vi "PC Main.vi"() -> ()   [LabVIEW 2018]
uses:
  <vilib>/Utility/inputDevices.llb/joystickAcquire.vi
  <vilib>/Utility/inputDevices.llb/closeJoystick.vi
  <resource>/objmgr/ni.dex.rc
panel:
  in  "myRIO IP address":string(combo)
  out "ScaledValues 2":dbl[](array[numeric])
  out "timed out?":bool
  in  "Stop Button":bool
  out "RT reader URL":string="//10.99.99.109/RT-reader"
  out "RT connected?":bool=TRUE
  out "error out 2":errorcluster
  out "direction info 3":T1={"pov 1"=-1, "pov 2"=-1, "pov 3"=-1, "pov 4"=-1}
  in  "stop 2":bool
  out "axis info 2":T2
  out "Angular Velocity":dbl
  out "Y velocity":dbl
  out "X velocity":dbl
  out "error out":errorcluster
  out "direction info 2":T1={"pov 1"=-1, "pov 2"=-1, "pov 3"=-1, "pov 4"=-1}
  in  "stop":bool
  out "array":i32[](array[numeric])=[289, 1907, -32768, 34, 2313, -32768, 0, 0]
  in  "LeftStick Deadzone -":dbl
  in  "LeftStick Deadzone +":dbl=2700.0
  in  "RightStick Deadzone -":dbl=-250.0
  in  "RightStick Deadzone +":dbl=2000.0
  out "LeftStick":dbl
  out "RightStick":dbl
  out "LeftOutput+":dbl
  out "LeftOutput-":dbl
  out "RightOutput+":dbl
  out "RightOutput-":dbl
  out "ScaledValues":dbl[](array[numeric])
  # "PC host writer"
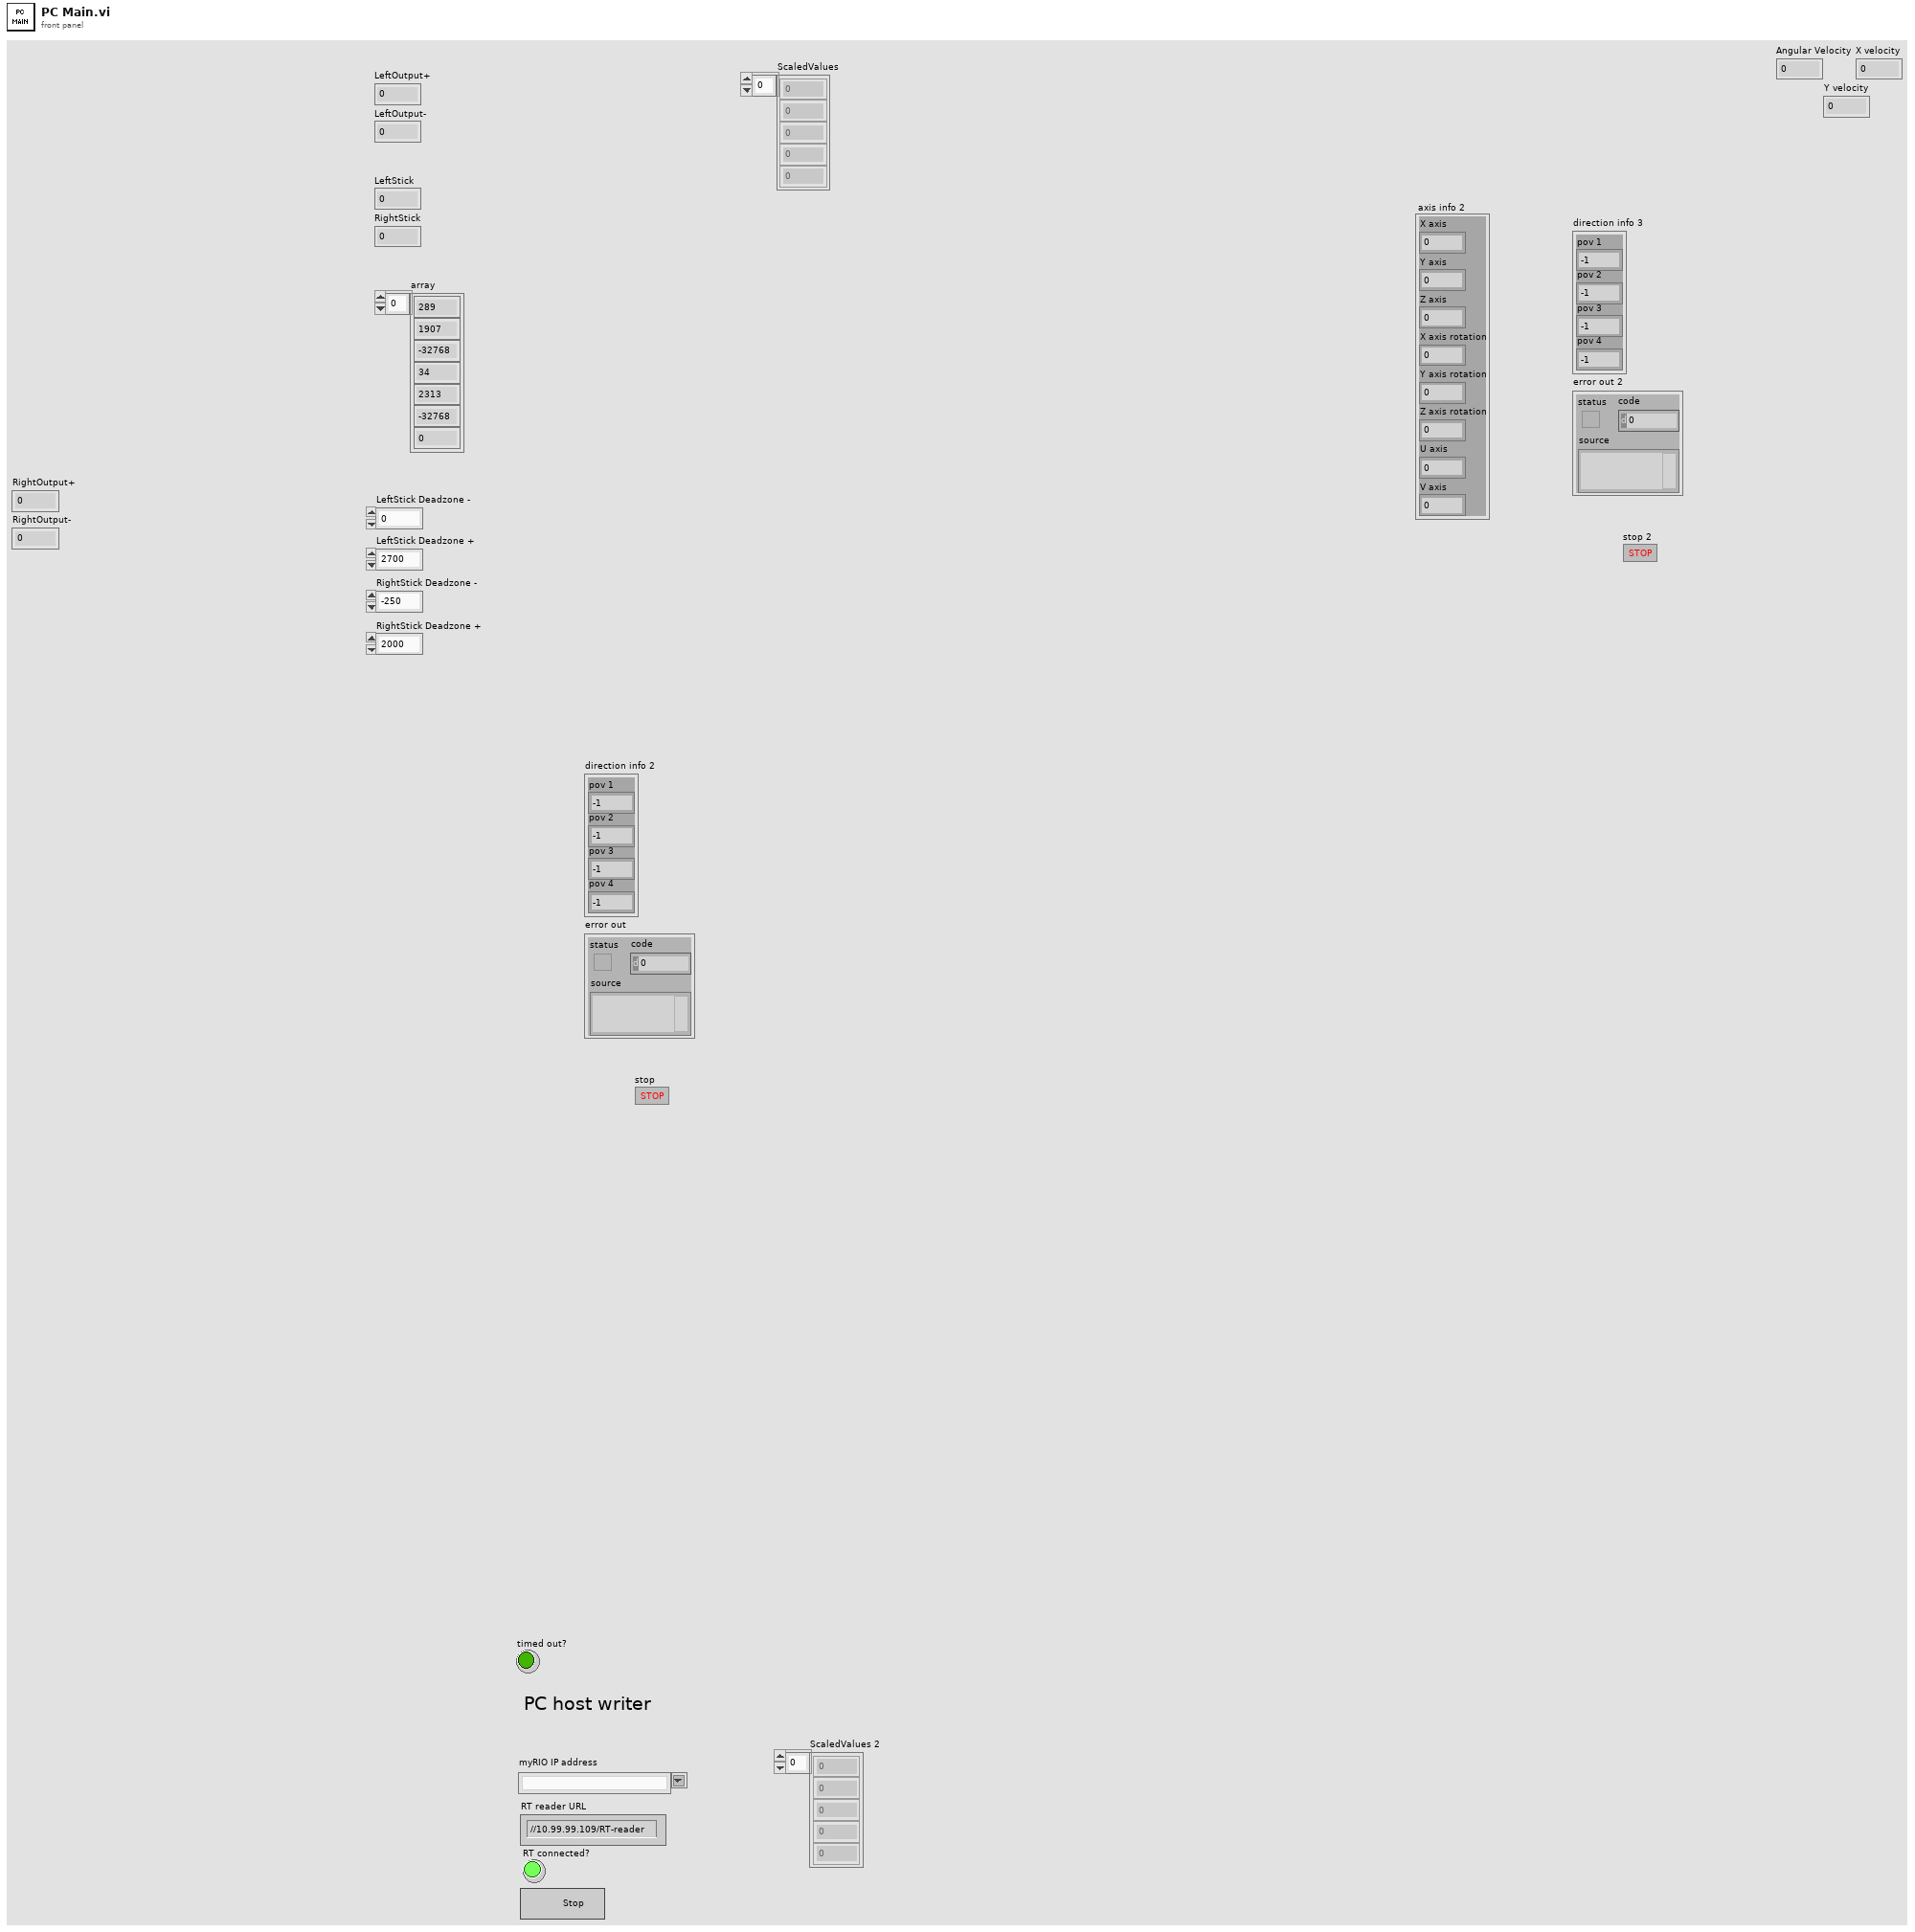
[diagram p1: front panel]
types:
  T1 = cluster{"pov 1":i32, "pov 2":i32, "pov 3":i32, "pov 4":i32}
  T2 = cluster{"X axis":i32, "Y axis":i32, "Z axis":i32, "X axis rotation":i32, "Y axis rotation":i32, "Z axis rotation":i32, "U axis":i32, "V axis":i32}
  T3 = cluster{"button 1":bool, "button 2":bool, "button 3":bool, "button 4":bool, "button 5":bool, "button 6":bool, "button 7":bool, "button 8":bool, "button 9":bool, "button 10":bool, "button 11":bool, "button 12":bool, "button 13":bool, "button 14":bool, "button 15":bool, "button 16":bool, "button 17":bool, "button 18":bool, "button 19":bool, "button 20":bool, "button 21":bool, "button 22":bool, "button 23":bool, "button 24":bool, "button 25":bool, "button 26":bool, "button 27":bool, "button 28":bool, "button 29":bool, "button 30":bool, "button 31":bool, "button 32":bool}
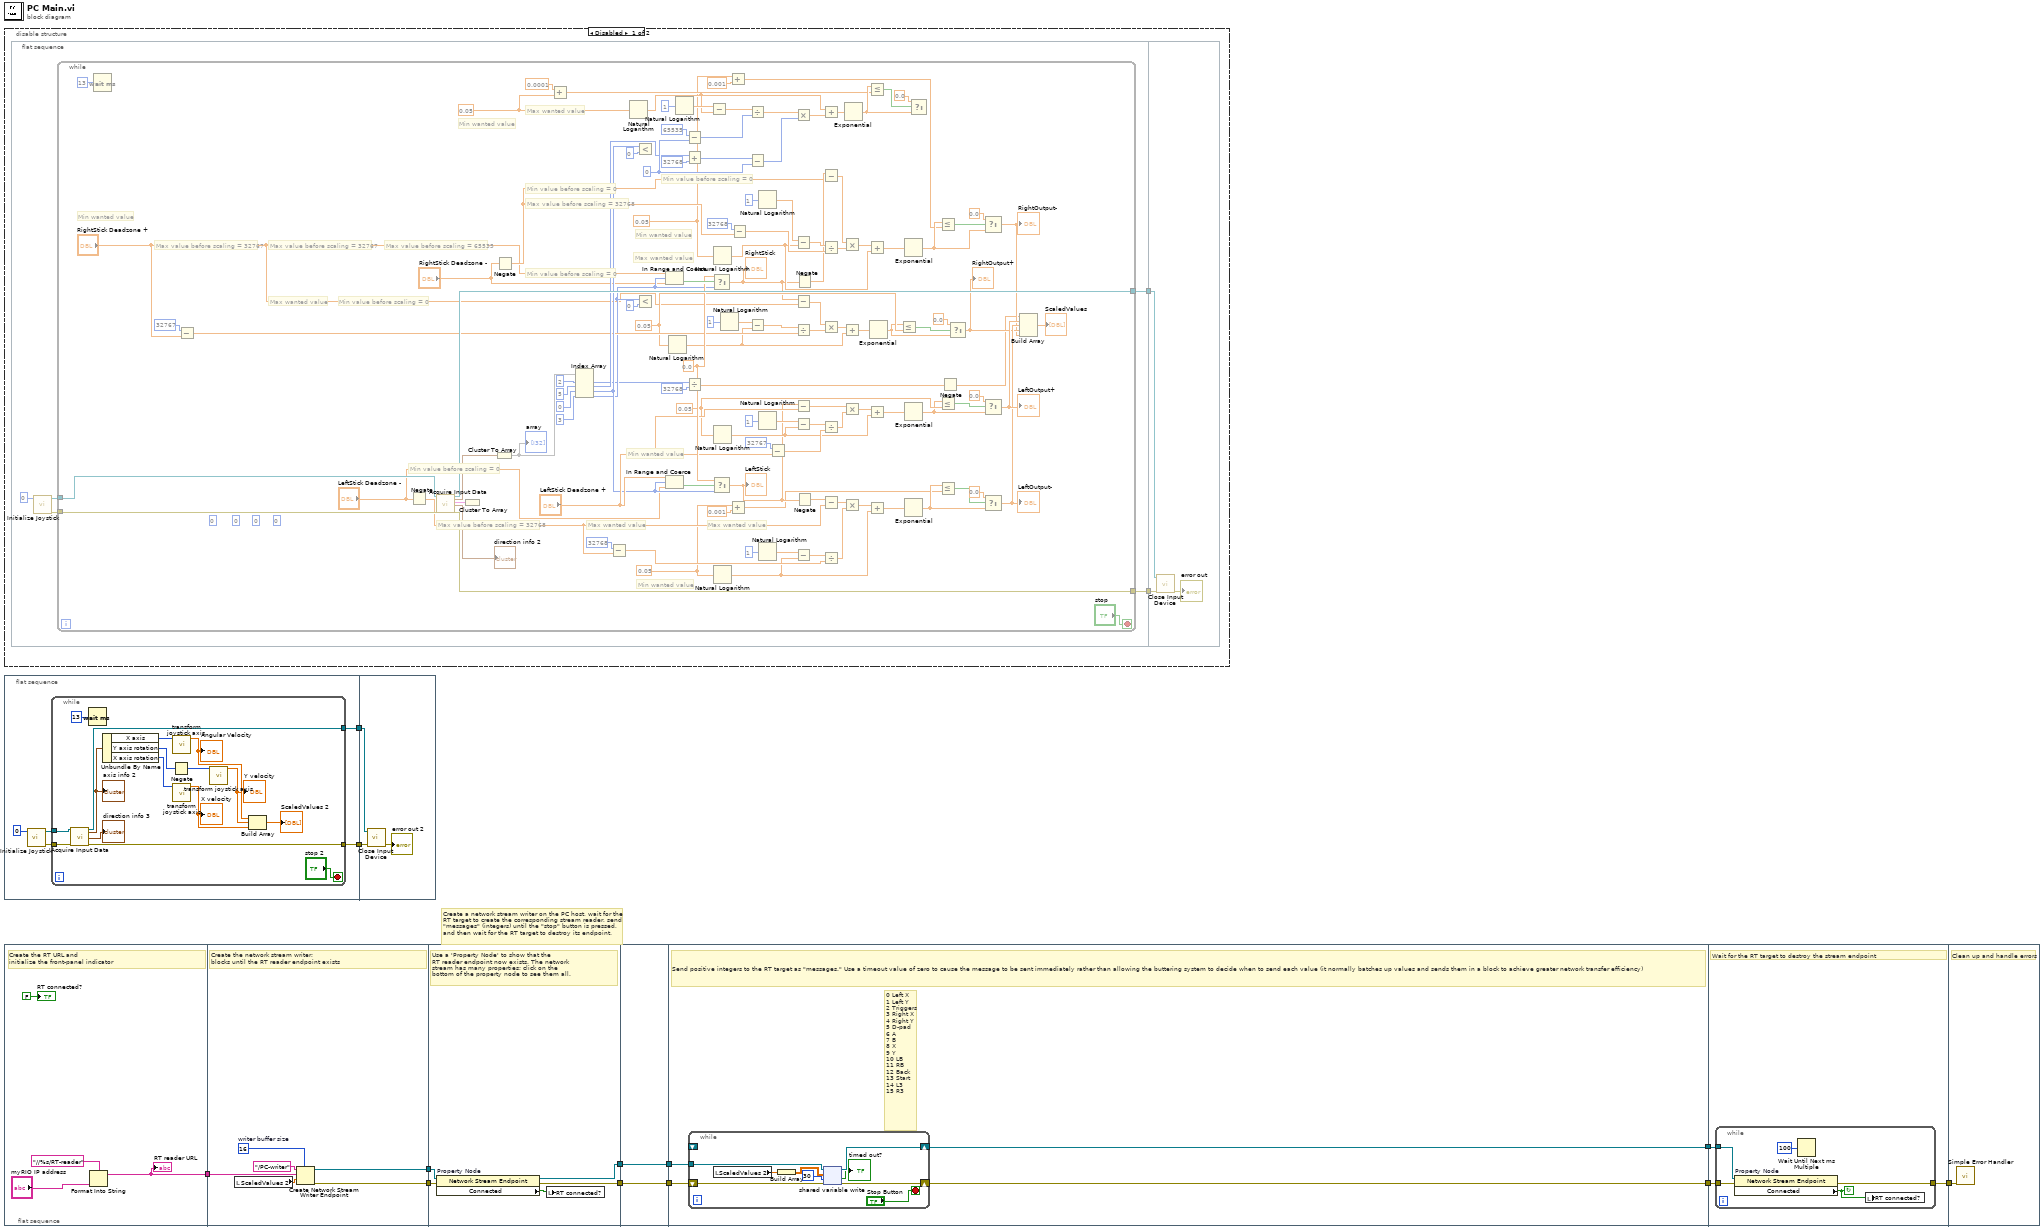
[diagram p0: block diagram]
diagram:
  # "Create a network stream writer on the PC host, wait for the\nRT target to create the corresponding stream reader, send\n\"messages\" (integers) until the \"stop\" button is pressed,\nand then wait for the RT target to destroy its endpoint."
  n1 = disable-structure shown="Disabled" {
    frame Disabled {
      n2 = flat-sequence {
        tunnel: [w17] -> w14
        tunnel: [w16] -> w13
        tunnel: w14 -> [w142]
        tunnel: w13 -> [w141]
        frame #0 {
          n3 = call <vilib>:"Initialize Joystick.vi"("device index"=0) -> ("error out"=w18:errorcluster, "device ID"=w19:refnum<k1>)  [unwired: 9 in]
          n4 = while {
            tunnel: w19 -> [w138]
            tunnel: w18 -> [w137]
            tunnel: [w136] -> w17
            tunnel: [w134] -> w16
            stop <- "stop" stop-if-true
            w35 = 0.05 ("x")
            (unwired) 0 ("index")
            w55 = 0.05 ("x")
            (unwired) 0 ("index")
            w68 = 0.05 ("x")
            (unwired) 0 ("index")
            w91 = 0.05 ("x")
            (unwired) 0 ("index")
            w103 = 0.0 ("t")
            w110 = 0.05 ("x")
            w124 = 0 ("index")
            # "Min wanted value"
            # "Max wanted value"
            # "Max value before scaling = 32768"
            # "Min value before scaling = 0"
            # "Min wanted value"
            # "Max wanted value"
            # "Max value before scaling = 32767"
            # "Min value before scaling = 0"
            # "Min wanted value"
            # "Max wanted value"
            # "Max value before scaling = 32768"
            # "Min value before scaling = 0"
            # "Min wanted value"
            # "Max wanted value"
            # "Max value before scaling = 32767"
            # "Min value before scaling = 0"
            # "Min wanted value"
            # "Max wanted value"
            # "Max value before scaling = 65535"
            # "Min value before scaling = 0"
            n5 = Wait (ms)(milliseconds to wait=u32 13) -> ()  [unwired: 1 out]
            n6 = Subtract(x=32767 ("index"), y="RightStick Deadzone +") -> (x-y=w61:dbl)
            n7 = Negate(x="LeftStick Deadzone -") -> (-x=w69:dbl)
            n8 = call-poly <vilib>:"Acquire Input Data.vi"("device ID"=w138, "error in (no error)"=w137) -> ("device ID"=w136:refnum<k1>, "axis info"=w133:T2, "button info"=w132:T3, "direction info"=→"direction info 2":T1, "error out"=w134:errorcluster)  [unwired: 13 in]
            n9 = Cluster To Array(cluster=w132) -> ()  [unwired: 1 out]
            n10 = Cluster To Array(cluster=w133) -> (array=w131:i32[])
            "array" <- w131
            n11 = Negate(x="RightStick Deadzone -") -> (-x=w36:dbl)
            n12 = Add(x=0.0001 ("y"), y=w110) -> (x+y=w108:dbl)
            n13 = Index Array(array=w131, index #1=2 ("index"), index #2=5 ("index"), index #3=0 ("index"), index #4=3 ("index")) -> (element #1=w22:i32, element #2=w116:i32, element #3=w73:i32, element #4=w32:i32)
            n14 = Subtract(x=32768 ("index"), y=w69) -> (x-y=w82:dbl)
            n15 = Natural Logarithm(1:w110) -> (0:w120:dbl)
            n16 = Less?(x=w73, y=0) -> ()  [unwired: 1 out]
            n17 = Less?(x=w32, y=0) -> ()  [unwired: 1 out]
            n18 = In Range and Coerce(upper limit="RightStick Deadzone +", x=w32, lower limit="RightStick Deadzone -") -> (In Range?=w105:bool)  [unwired: 1 out]
            n19 = In Range and Coerce(upper limit="LeftStick Deadzone +", x=w73, lower limit="LeftStick Deadzone -") -> (In Range?=w104:bool)  [unwired: 1 out]
            n20 = Natural Logarithm(1:w55) -> (0:w57:dbl)
            n21 = Natural Logarithm(1:1 ("index")) -> (0:w128:dbl)
            n22 = Subtract(x=65535 ("index"), y=w124) -> (x-y=w125:i32)
            n23 = Add(x=w116, y=32768) -> (x+y=w115:i32)
            n24 = Divide(x=w22, y=32768) -> (x/y=w21:dbl)
            n25 = Subtract(x=w128, y=w120) -> (x-y=w127:dbl)
            n26 = Select(t=w103, s=w105, f=w32) -> (s? t:f=w31:dbl)
            "RightStick" <- w31
            n27 = Select(t=w103, s=w104, f=w73) -> (s? t:f=w72:dbl)
            "LeftStick" <- w72
            n28 = Natural Logarithm(1:w35) -> (0:w42:dbl)
            n29 = Natural Logarithm(1:w91) -> (0:w93:dbl)
            n30 = Natural Logarithm(1:w68) -> (0:w78:dbl)
            n31 = Natural Logarithm(1:1 ("index")) -> (0:w63:dbl)
            n32 = Add(x=w35, y=0.001) -> (x+y=w33:dbl)
            n33 = Add(x=w68, y=0.001) -> (x+y=w66:dbl)
            n34 = Subtract(x=32768 ("index"), y=w36) -> (x-y=w46:dbl)
            n35 = Divide(x=w127, y=w125) -> (x/y=w122:dbl)
            n36 = Subtract(x=w115, y=w124) -> (x-y=w123:i32)
            n37 = Subtract(x=w63, y=w57) -> (x-y=w62:dbl)
            n38 = Natural Logarithm(1:1 ("index")) -> (0:w48:dbl)
            n39 = Natural Logarithm(1:1 ("index")) -> (0:w100:dbl)
            n40 = Natural Logarithm(1:1 ("index")) -> (0:w84:dbl)
            n41 = Subtract(x=32767 ("index"), y="LeftStick Deadzone +") -> (x-y=w98:dbl)
            n42 = Multiply(x=w122, y=w123) -> (x*y=w121:dbl)
            n43 = Subtract(x=w48, y=w42) -> (x-y=w47:dbl)
            n44 = Subtract(x=w31, y="RightStick Deadzone +") -> (x-y=w60:dbl)
            n45 = Divide(x=w62, y=w61) -> (x/y=w59:dbl)
            n46 = Subtract(x=w72, y="LeftStick Deadzone +") -> (x-y=w96:dbl)
            n47 = Subtract(x=w100, y=w93) -> (x-y=w99:dbl)
            n48 = Subtract(x=w84, y=w78) -> (x-y=w83:dbl)
            n49 = Negate(x=w31) -> (-x=w37:dbl)
            n50 = Negate(x=w72) -> (-x=w71:dbl)
            n51 = Add(x=w120, y=w121) -> (x+y=w119:dbl)
            n52 = Subtract(x=w37, y=w36) -> (x-y=w45:dbl)
            n53 = Divide(x=w47, y=w46) -> (x/y=w44:dbl)
            n54 = Multiply(x=w60, y=w59) -> (x*y=w58:dbl)
            n55 = Divide(x=w99, y=w98) -> (x/y=w95:dbl)
            n56 = Subtract(x=w71, y=w69) -> (x-y=w81:dbl)
            n57 = Divide(x=w83, y=w82) -> (x/y=w80:dbl)
            n58 = Multiply(x=w45, y=w44) -> (x*y=w43:dbl)
            n59 = Add(x=w58, y=w57) -> (x+y=w56:dbl)
            n60 = Multiply(x=w96, y=w95) -> (x*y=w94:dbl)
            n61 = Multiply(x=w81, y=w80) -> (x*y=w79:dbl)
            n62 = Exponential(1:w119) -> (0:w111:dbl)
            n63 = Less Or Equal?(x=w111, y=w108) -> (x <= y?=w113:bool)
            n64 = Add(x=w43, y=w42) -> (x+y=w41:dbl)
            n65 = Add(x=w94, y=w93) -> (x+y=w92:dbl)
            n66 = Add(x=w79, y=w78) -> (x+y=w77:dbl)
            n67 = Exponential(1:w56) -> (0:w52:dbl)
            n68 = Less Or Equal?(x=w52, y=w55) -> (x <= y?=w54:bool)
            n69 = Exponential(1:w41) -> (0:w38:dbl)
            n70 = Exponential(1:w92) -> (0:w88:dbl)
            n71 = Exponential(1:w77) -> (0:w74:dbl)
            n72 = Select(t=0.0, s=w113, f=w111) -> ()  [unwired: 1 out]
            n73 = Less Or Equal?(x=w38, y=w33) -> (x <= y?=w40:bool)
            n74 = Less Or Equal?(x=w88, y=w91) -> (x <= y?=w90:bool)
            n75 = Less Or Equal?(x=w74, y=w66) -> (x <= y?=w76:bool)
            n76 = Negate(x=w21) -> (-x=w20:dbl)
            n77 = Select(t=0.0, s=w54, f=w52) -> (s? t:f=w25:dbl)
            "RightOutput+" <- w25
            n78 = Select(t=0.0, s=w40, f=w38) -> (s? t:f=w24:dbl)
            "RightOutput-" <- w24
            n79 = Select(t=0.0, s=w90, f=w88) -> (s? t:f=w27:dbl)
            "LeftOutput+" <- w27
            n80 = Select(t=0.0, s=w76, f=w74) -> (s? t:f=w26:dbl)
            "LeftOutput-" <- w26
            n81 = Build Array(w20, w27, w26, w25, w24) -> (→"ScaledValues":dbl[])
          }
        }
        frame #1 {
          n82 = call-poly <vilib>:"Close Input Device.vi"("error in (no error)"=w141, "device ID"=w142) -> ("error out"=→"error out":errorcluster)  [unwired: 8 in]
        }
      }
    }
    frame Enabled {
    }
  }
  n83 = flat-sequence {
    tunnel: [w145] -> w2
    tunnel: [w144] -> w1
    tunnel: w2 -> [w166]
    tunnel: w1 -> [w165]
    frame #0 {
      n84 = call <vilib>:"Initialize Joystick.vi"("device index"=0) -> ("error out"=w146:errorcluster, "device ID"=w147:refnum<k1>)  [unwired: 9 in]
      n85 = while {
        tunnel: w147 -> [w162]
        tunnel: w146 -> [w161]
        tunnel: [w160] -> w145
        tunnel: [w158] -> w144
        stop <- "stop 2" stop-if-true
        n86 = call-poly <vilib>:"Acquire Input Data.vi"("device ID"=w162, "error in (no error)"=w161) -> ("device ID"=w160:refnum<k1>, "axis info"=w156:T2, "direction info"=→"direction info 3":T1, "error out"=w158:errorcluster)  [unwired: 13 in, 1 out]
        "axis info 2" <- w156
        n87 = Wait (ms)(milliseconds to wait=u32 13) -> ()  [unwired: 1 out]
        n88 = Unbundle By Name(w156) -> ("X axis"=w154:i32, "Y axis rotation"=w155:i32, "X axis rotation"=w152:i32)
        n89 = Negate(x=w155) -> (-x=w153:i32)
        n90 = call <vilib>:"transform joystick axis.vi"("Axis Input"=w154) -> ("Output (-1..1)"=w151:dbl)  [unwired: 10 in]
        "Angular Velocity" <- w151
        n91 = call <vilib>:"transform joystick axis.vi"("Axis Input"=w152) -> ("Output (-1..1)"=w149:dbl)  [unwired: 10 in]
        "X velocity" <- w149
        n92 = call <vilib>:"transform joystick axis.vi"("Axis Input"=w153) -> ("Output (-1..1)"=w150:dbl)  [unwired: 10 in]
        "Y velocity" <- w150
        n93 = Build Array(w151, w150, w149) -> (→"ScaledValues 2":dbl[])
      }
    }
    frame #1 {
      n94 = call-poly <vilib>:"Close Input Device.vi"("error in (no error)"=w165, "device ID"=w166) -> ("error out"=→"error out 2":errorcluster)  [unwired: 8 in]
    }
  }
  n95 = flat-sequence {
    tunnel: [w169] -> w12
    tunnel: w12 -> [w174]
    tunnel: [w173] -> w11
    tunnel: [w172] -> w10
    tunnel: w11 -> [w181]
    tunnel: w10 -> [w180]
    tunnel: [w179] -> w6
    tunnel: [w178] -> w4
    tunnel: w6 -> [w183]
    tunnel: [w183] -> w5
    tunnel: w4 -> [w182]
    tunnel: [w182] -> w3
    tunnel: w5 -> [w187]
    tunnel: w3 -> [w186]
    tunnel: [w185] -> w9
    tunnel: [w184] -> w8
    tunnel: w9 -> [w199]
    tunnel: w8 -> [w198]
    tunnel: [w197] -> w7
    tunnel: w7 -> [w205]
    frame #0 {
      # "Create the RT URL and\ninitialize the front-panel indicator"
      n96 = Format Into String "Format Into String"(format string="//%s/RT-reader", "myRIO IP address") -> (resulting string=w169:string)  [unwired: 2 in, 1 out]
      "RT reader URL" <- w169
      "RT connected?" <- FALSE ("RT connected?")
    }
    frame #1 {
      w176 = 16  # writer buffer size
      # "Create the network stream writer;\nblocks until the RT reader endpoint exists"
      n97 = local read "ScaledValues 2"() -> (w171:dbl[])
      n98 = Create Network Stream Writer Endpoint(7:w176, 9:w171, 10:w174, 11:"/PC-writer" ("writer name")) -> (0:w172:errorcluster, 3:w173:refnum<k21>)  [unwired: 3 in]
    }
    frame #2 {
      # "Use a 'Property Node' to show that the\nRT reader endpoint now exists. The network\nstream has many properties; click on the\nbottom of the property node to see them all."
      n99 = property on="Property Node" class="Network Stream Endpoint"(reference=w181, error in=w180) -> (reference out=w179:refnum<k21>, error out=w178:errorcluster, "Connected"=w177:bool)
      n100 = local write "RT connected?"(w177) -> ()
    }
    frame #3 {
    }
    frame #4 {
      # "0 Left X\n1 Left Y\n2 Triggers\n3 Right X\n4 Right Y\n5 D-pad\n6 A\n7 B\n8 X\n9 Y\n10 LB\n11 RB\n12 Back\n13 Start\n14 L3\n15 R3"
      # "Send positive integers to the RT target as \"messages.\" Use a timeout value of zero to cause the message to be sent immediately rather than allowing the buttering system to decide when to send each value (it normally batches up values and sends them in a block to achieve greater network transfer efficiency)"
      n101 = while {
        shift-right: [w192] -> w184
        shift-left: w186 -> [w193]
        tunnel: w187 -> [w195]
        shift-right: [w191] -> w185
        shift-left: _ -> [_]
        stop <- "Stop Button" stop-if-true
        n102 = local read "ScaledValues 2"() -> (w189:dbl[])
        n103 = Build Array(w189) -> (w188:dbl[][])
        n104 = shared-variable-write(w195, w193, w188, 30 ("timeout ms (-1)")) -> (w191:refnum<k21>, w192:errorcluster, →"timed out?":bool)
      }
    }
    frame #5 {
      # "Wait for the RT target to destroy the stream endpoint"
      n105 = while {
        tunnel: w199 -> [w204]
        tunnel: w198 -> [w203]
        tunnel: [w202] -> w197
        stop <- w200 continue-if-true
        # "wait for RT to destroy the endpoint"
        n106 = property on="Property Node" class="Network Stream Endpoint"(reference=w204, error in=w203) -> (error out=w202:errorcluster, "Connected"=w200:bool)  [unwired: 1 out]
        n107 = Wait Until Next ms Multiple(millisecond multiple=u32 100) -> ()  [unwired: 1 out]
        n108 = local write "RT connected?"(w200) -> ()
      }
    }
    frame #6 {
      # "Clean up and handle errors"
      n109 = call <vilib>:"Simple Error Handler.vi"("error in (no error)"=w205) -> ()  [unwired: 4 in, 5 out]
    }
  }
